vi "Clear.vi"(3 "((Pointer)) in":refnum<class "_Pointer.lvclass">) -> (1 "((Pointer)) out":refnum<class "_Pointer.lvclass">)   [LabVIEW 2025, in "_Pointer.lvclass"]
uses:
  _Pointer.lvclass
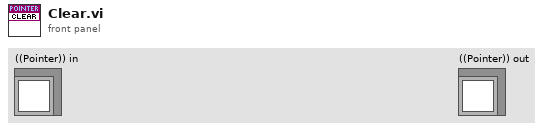
[diagram p1: front panel]
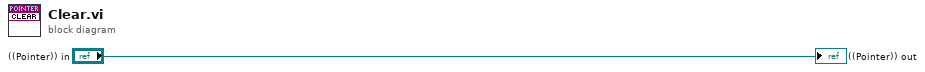
[diagram p0: block diagram]
diagram:
  "((Pointer)) out" <- "((Pointer)) in"
